vi "Get Dimension.vi"(8 "error in (no error)":errorcluster, 11 "Signal in":refnum<class "Signal.lvclass">) -> (0 "error out":errorcluster, 2 "Ending out":refnum<class "Data.lvclass">, 3 "Signal out":refnum<class "Signal.lvclass">)   [LabVIEW 2013, in "MDSplus.lvlib" / "Signal.lvclass"]
uses:
  <vilib>/MDSplus/Classes/Data_Class/Compound_Class/Signal_Class/Signal.lvclass
  <vilib>/MDSplus/Classes/Data_Class/Data.lvclass
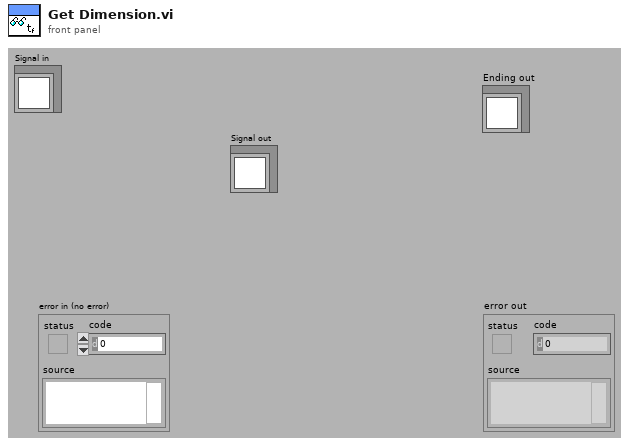
[diagram p1: front panel]
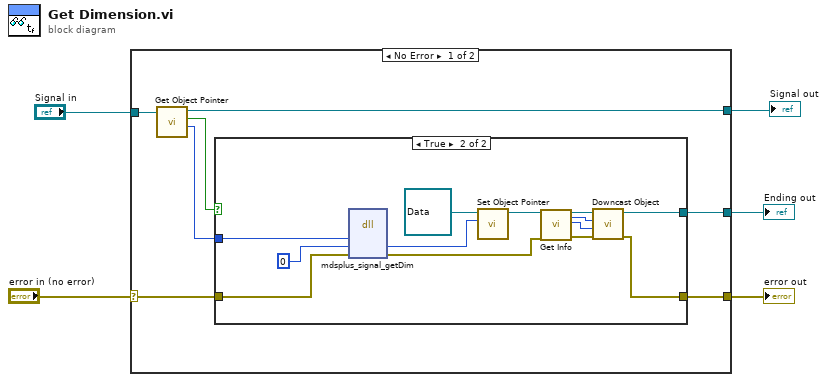
[diagram p0: block diagram]
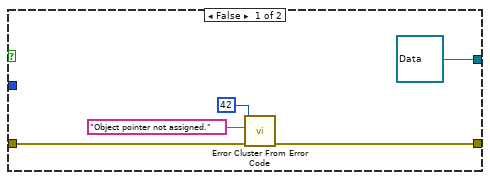
[diagram p2: hidden frame]
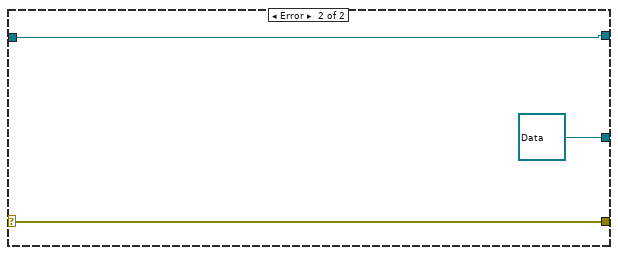
[diagram p3: hidden frame]
diagram:
  n1 = case shown="No Error" "error in (no error)" {
    selector: "error in (no error)" -> [w9 w33]
    tunnel: [w8 w33] -> w4
    tunnel: [w7 w31] -> w1
    tunnel: [w12 refnum<class "Data.lvclass"> refnum ("Data out")] -> w3
    tunnel: "Signal in" -> [w6 w31]
    frame No Error {
      n2 = call-dynamic "Get Object Pointer.vi"("Data in"=w6) -> ("Object Pointer"=w10:i64, "Assigned object pointer?"=w11:bool, "Data out"=w7:refnum<class "Signal.lvclass">)  [unwired: 8 in]
      n3 = case shown="True" w11 {
        tunnel: [refnum<class "Data.lvclass"> refnum ("Data out") w22] -> w12
        tunnel: w10 -> [_ w21]
        tunnel: w9 -> [w14 w19]
        tunnel: [w13 w18] -> w8
        frame False {
          n4 = call <vilib>:"Error Cluster From Error Code.vi"("error in (no error)"=w14, "error message (\"\")"="Object pointer not assigned." ("error message (\"\")"), "error code (0)"=42) -> ("error out"=w13:errorcluster)  [unwired: 6 in]
        }
        frame True {
          n5 = dll-call lib="MDSobjectsLVShr" fn="mdsplus_signal_getDim"("lvSignalPtr"=w21, "lvDim0PtrOut"=i64 0 ("lvDataPtrOut"), "error"=w19) -> ("lvDim0PtrOut"=w28:i64, "error"=w20:errorcluster)  [unwired: 5 in, 2 out]
          n6 = call-dynamic "Set Object Pointer.vi"("Object Pointer"=w28, "Data in"=refnum<class "Data.lvclass"> refnum ("Data.lvclass")) -> ("Data out"=w27:refnum<class "Data.lvclass">)  [unwired: 9 in]
          n7 = call-dynamic "Get Info.vi"("Data in"=w27, "error in (no error)"=w20) -> ("Data out"=w26:refnum<class "Data.lvclass">, "Class type out"=w25:u8, "Data type out"=w24:u8, "error out"=w23:errorcluster)  [unwired: 12 in, 2 out]
          n8 = call <vilib>:"Downcast Object.vi"("error in (no error)"=w23, "Data Type"=w24, "Class Type"=w25, "Data in"=w26) -> ("error out"=w18:errorcluster, "Data out"=w22:refnum<class "Data.lvclass">)  [unwired: 6 in]
        }
      }
    }
    frame Error {
    }
  }
  "error out" <- w4
  "Ending out" <- w3
  "Signal out" <- w1
